vi "BlendAlphaColor.vi"(9 "Alpha [0..1]":dbl, 10 "BG Color Component":u8, 11 "Image Color Component":u8) -> (3 "New Image Color":u8)   [LabVIEW 2020, in "lv-image.lvlib"]
uses:
  lv-image.lvlib
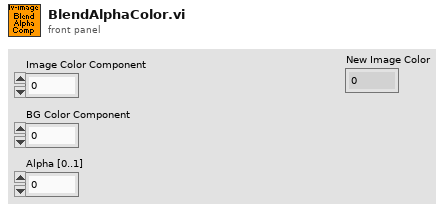
[diagram p1: front panel]
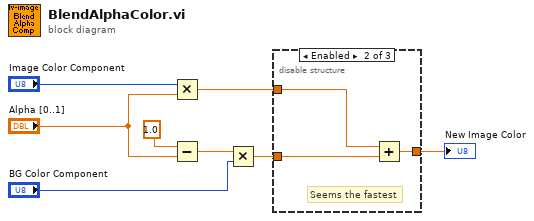
[diagram p0: block diagram]
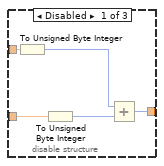
[diagram p2: hidden frame]
diagram:
  n1 = Multiply(x="Image Color Component", y="Alpha [0..1]") -> (x*y=w3:dbl)
  n2 = Subtract(x=1.0, y="Alpha [0..1]") -> (x-y=w5:dbl)
  n3 = Multiply(x=w5, y="BG Color Component") -> (x*y=w2:dbl)
  n4 = disable-structure shown="Enabled" {
    disable-tunnel: w3 -> [w13 w14 _]
    disable-tunnel: w2 -> [w12 w16 _]
    disable-tunnel: [w11 w15 _] -> w1
    frame Disabled {
      n5 = To Unsigned Byte Integer(number=w13) -> (unsigned 8bit integer=w10:u8)
      n6 = To Unsigned Byte Integer(number=w12) -> (unsigned 8bit integer=w9:u8)
      n7 = Add(x=w10, y=w9) -> (x+y=w11:u8)
    }
    frame Enabled {
      # "Seems the fastest"
      n8 = Add(x=w14, y=w16) -> (x+y=w15:dbl)
    }
    frame Disabled {
    }
  }
  "New Image Color" <- w1
